vi "Actor Core.vi"(8 "error in":errorcluster, 11 "Game Engine in":refnum<class "Game Engine.lvclass">) -> (0 "error out":errorcluster, 3 "Actor out":refnum<class "Actor.lvclass">)   [LabVIEW 2017, in "Game Engine.lvlib" / "Game Engine.lvclass"]
doc: "(<B>Filename</B>: Actor Framework.lvlib:Actor.lvclass:Actor Core.vi)\n\nReceives messages to the actor, reacts to them, and initiates any error handling that may shut the actor down.\n\nDescendant classes may override this VI to append parallel tasks for the actor to complete while it handles messages. Overrides use the Call Parent Method node."
uses:
  Game Engine.lvclass
  <vilib>/ActorFramework/Actor/Actor.lvclass
  Simulated Screen Interface/Simulated Screen Interface/Simulated Screen Interface.lvclass
  C:/Program Files (x86)/National Instruments/LabVIEW 2017/vi.lib/ActorFramework/Actor/Actor.lvclass
  Simulated Game Pad Interface/Simulated Game Pad Interface.lvclass
  C:/Users/chris/Documents/GitHub/Tetris/RT Code/Abstract Game Pad Interface/Abstract Game Pad Interface.lvclass
  Simulated Screen Interface/Simulated Screen Interface Messages/Update Display Msg/Update Display Msg.lvclass
  C:/Users/chris/Documents/GitHub/Tetris/RT Code/Screen Interface/Screen Interface Messages/Display Game Board Msg/Display Game Board Msg.lvclass
  Game Engine.lvclass/Game Engine.ctl
  <vilib>/Platform/TimedLoop/XDataNode/timing_clust.ctl
  <vilib>/Platform/TimedLoop/XDataNode/nitl_modes.ctl
  <vilib>/Platform/TimedLoop/XDataNode/wakeup.ctl
  Error Handler/Error Handler/Error Handler.lvclass
  <vilib>/Platform/TimedLoop/XDataNode/XDataNode.xnode
  Abstract Game Pad Interface/Abstract Game Pad Interface.lvclass
  <vilib>/Platform/TimedLoop/XDataNode/XDNodeRunTimeDep.lvlib
  Hardware Game Pad Interface/Hardware Game Pad Interface.lvclass
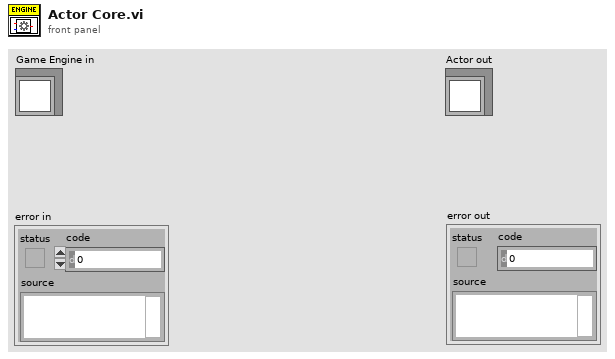
[diagram p1: front panel]
types:
  T1 = typedef "XDNodeRunTimeDep.lvlib/timing_clust.ctl" = cluster{"Expected End [f-1]":u64, "Actual End [f-1]":u64, "Finished Late? [f-1]":bool, "Expected End [i-1]":u64, "Actual End [i-1]":u64, "Finished Late? [i-1]":bool, "Expected Start [i]":u64, "Actual Start [i]":u64, "Expected Start [f]":u64, "Actual Start [f]":u64, "Source Name":string, "Structure Name":string, "Period":i64, "Deadline":i64, "Offset":i64, "Start":i64, "Priority":i32, "Timeout":i32, "Mode":T2, "Wakeup Reason":T3, "Error":errorcluster, "Source Type":string, "Secondary Source Type":string, "Global End Time":u64, "Global Start Time":u64, "Frame Duration":u64, "Iteration Duration":u64, "Assigned CPU":i32, "I/O Scan Engine Mode":u32}
  T2 = typedef "XDNodeRunTimeDep.lvlib/nitl_modes.ctl" = enum32{"No Change", "Process missed periods, maintain original phase", "Discard missed periods, maintain original phase", "Process missed periods, ignore original phase", "Discard missed periods, ignore original phase"}
  T3 = typedef "XDNodeRunTimeDep.lvlib/wakeup.ctl" = enum32{"Normal", "Aborted", "Asynchronous wakeup", "Timing source error", "Timed loop error", "Timeout"}
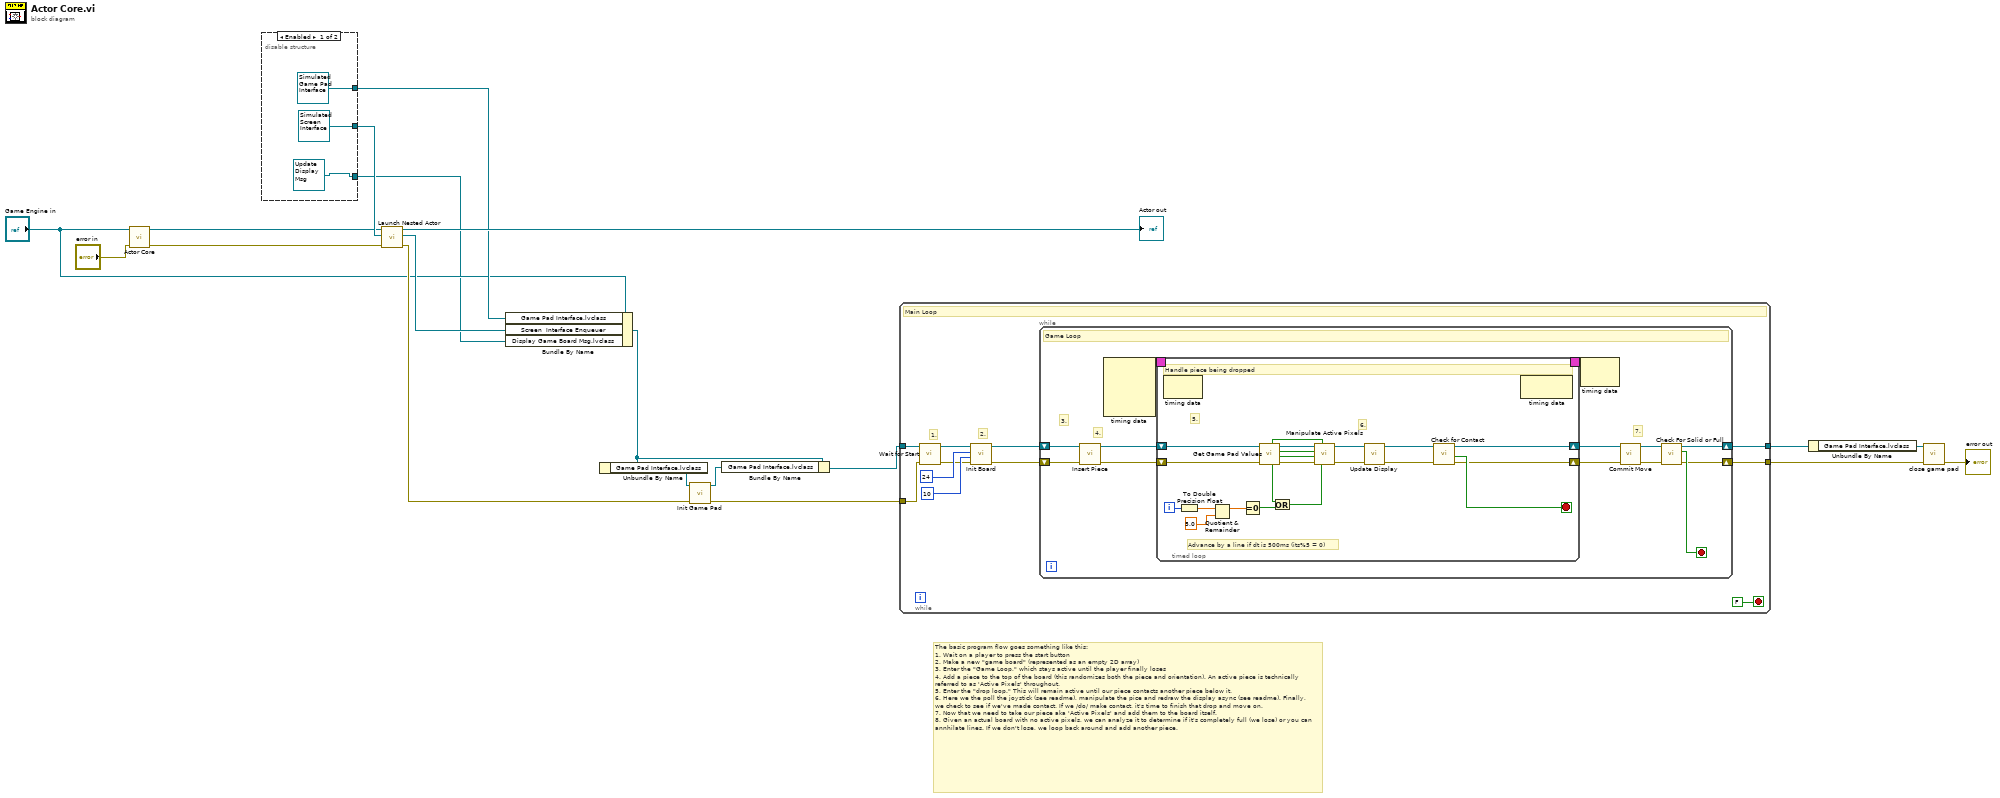
[diagram p0: block diagram]
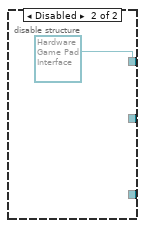
[diagram p2: hidden frame]
diagram:
  # "The basic program flow goes something like this:\n1. Wait on a player to press the start button\n2. Make a new \"game board\" (represented as an empty 2D array)\n3. Enter the \"Game Loop,\" which stays active until the player finally loses\n4. Add a piece to the top of the board (this randomizes both the piece and orientation). An active piece is technically referred to as 'Active Pixels' throughout.\n5. Enter the \"drop loop.\" This will remain active until our piece contacts another piece below it.\n6. Here we the poll the joystick (see readme), manipulate the pice and redraw the display async (see readme). Finally, we check to see if we've made contact. If we /do/ make contact, it's time to finish that drop and move on.\n7. Now that we need to take our piece aka 'Active Pixels' and add them to the board itself. \n8. Given an actual board with no active pixels, we can analyze it to determine if it's completely full (we lose) or you can annhilate lines. If we don't lose, we loop back around and add another piece."
  n1 = call-parent "Actor Core.vi"("error in"="error in", "Controller in"="Game Engine in") -> ("error out"=w3:errorcluster, "Actor out"=w6:refnum<class "Actor.lvclass">)  [unwired: 8 in]
  n2 = disable-structure shown="Enabled" {
    disable-tunnel: [refnum<class "Simulated Screen Interface.lvclass"> refnum ("Simulated Screen Interface.lvlib:Simulated Screen Interface.lvclass") w24] -> w19
    disable-tunnel: [refnum<class "Simulated Game Pad Interface.lvclass"> refnum ("Simulated Game Pad Interface.lvclass") refnum<class "Hardware Game Pad Interface.lvclass"> refnum ("Hardware Game Pad Interface.lvclass")] -> w15
    disable-tunnel: [refnum<class "Update Display Msg.lvclass"> refnum ("Simulated Screen Interface.lvlib:Update Display Msg.lvclass") w23] -> w1
    frame Enabled {
    }
    frame Disabled {
    }
  }
  n3 = call <vilib>:"Launch Nested Actor.vi"("error in (no error)"=w3, "Nested Actor"=w19, "Caller Actor in"=w6) -> ("error out"=w16:errorcluster, "Nested Actor's Enqueuer"=w18:refnum<class "Message Enqueuer.lvclass">, "Caller Actor out"=→"Actor out":refnum<class "Actor.lvclass">)  [unwired: 6 in]
  n4 = Bundle By Name(cluster="Game Engine in", "Game Pad Interface.lvclass"=w15, "Screen  Interface Enqueuer"=w18, "Display Game Board Msg.lvclass"=w1) -> (w13:refnum<class "Game Engine.lvclass">)
  n5 = Unbundle By Name(w13) -> ("Game Pad Interface.lvclass"=w14:refnum<class "Abstract Game Pad Interface.lvclass">)
  n6 = call-dynamic "Init Game Pad.vi"("error in (no error)"=w16, "Abstract Game Pad Interface in"=w14) -> ("error out"=w10:errorcluster, "Abstract Game Pad Interface out"=w12:refnum<class "Abstract Game Pad Interface.lvclass">)  [unwired: 8 in]
  n7 = Bundle By Name(cluster=w13, "Game Pad Interface.lvclass"=w12) -> (w11:refnum<class "Game Engine.lvclass">)
  n8 = while {
    tunnel: w11 -> [w32]
    tunnel: [w28] -> w7
    tunnel: [w27] -> w9
    tunnel: w10 -> [w26]
    stop <- FALSE stop-if-true
    # "2."
    # "1."
    # "Main Loop"
    n9 = call "Wait for Start.vi"("error in (no error)"=w26, "Game Engine in"=w32) -> ("error out"=w30:errorcluster, "Game Engine out"=w31:refnum<class "Game Engine.lvclass">)  [unwired: 8 in]
    n10 = call "Init Board.vi"("error in (no error)"=w30, "Columns"=u8 10, "Rows"=u8 24, "Game Engine in"=w31) -> ("error out"=w33:errorcluster, "Game Engine out"=w34:refnum<class "Game Engine.lvclass">)  [unwired: 6 in]
    n11 = while {
      shift-right: [w37] -> w27
      shift-left: w34 -> [w47]
      shift-right: [w38] -> w28
      shift-left: w33 -> [w46]
      stop <- w39 stop-if-true
      # "7."
      # "4."
      # "3."
      # "Game Loop"
      n12 = call "Insert Piece.vi"("error in (no error)"=w46, "Game Engine in"=w47) -> ("error out"=w44:errorcluster, "Game Engine out"=w45:refnum<class "Game Engine.lvclass">)  [unwired: 8 in]
      n13 = node-c288() -> (w49:T1)  [unwired: 4 in]
      n14 = timed-loop {
        timing: w49 -> [_]
        timing-out: [_] -> w48
        shift-right: [w50] -> w43
        shift-left: w45 -> [w57]
        shift-right: [w51] -> w42
        shift-left: w44 -> [w56]
        i -> [w69]
        stop <- w70 stop-if-true
        # "6."
        # "5."
        # "Advance by a line if dt is 500ms (its%5 = 0)"
        # "Handle piece being dropped"
        n15 = node-c288() -> ()  [unwired: 1 in, 1 out]
        n16 = To Double Precision Float(number=w69) -> (double precision float=w68:dbl)
        n17 = Quotient & Remainder(x=w68, y=5.0) -> (x-y*floor(x/y)=w66:dbl)  [unwired: 1 out]
        n18 = Equal To 0?(x=w66) -> (x = 0?=w65:bool)
        n19 = call "Get Game Pad Values.vi"("error in (no error)"=w56, "Game Engine in"=w57) -> ("error out"=w60:errorcluster, "Right"=w61:bool, "Left"=w62:bool, "Game Engine out"=w59:refnum<class "Game Engine.lvclass">, "Down"=w64:bool, "Rotate"=w58:bool)  [unwired: 3 in, 1 out]
        n20 = Or(x=w64, y=w65) -> (x .or. y?=w63:bool)
        n21 = call "Manipulate Active Pixels.vi"("Advance Line"=w63, "Rotate"=w58, "error in (no error)"=w60, "Right"=w61, "Left"=w62, "Game Engine in"=w59) -> ("error out"=w54:errorcluster, "Game Engine out"=w55:refnum<class "Game Engine.lvclass">)  [unwired: 4 in]
        n22 = call "Update Display.vi"("error in (no error)"=w54, "Game Engine in"=w55) -> ("error out"=w53:errorcluster, "Game Engine out"=w52:refnum<class "Game Engine.lvclass">)  [unwired: 8 in]
        n23 = call "Check for Contact.vi"("error in (no error)"=w53, "Game Engine in"=w52) -> ("error out"=w51:errorcluster, "Contact"=w70:bool, "Game Engine out"=w50:refnum<class "Game Engine.lvclass">)  [unwired: 7 in]
        n24 = node-c288() -> ()  [unwired: 1 in, 1 out]
      }
      n25 = node-c288(w48) -> ()  [unwired: 1 out]
      n26 = call "Commit Move.vi"("error in (no error)"=w42, "Game Engine in"=w43) -> ("error out"=w40:errorcluster, "Game Engine out"=w41:refnum<class "Game Engine.lvclass">)  [unwired: 8 in]
      n27 = call "Check For Solid or Full.vi"("error in (no error)"=w40, "Game Engine in"=w41) -> ("error out"=w38:errorcluster, "Game Over"=w39:bool, "Game Engine out"=w37:refnum<class "Game Engine.lvclass">)  [unwired: 7 in]
    }
  }
  n28 = Unbundle By Name(w9) -> ("Game Pad Interface.lvclass"=w8:refnum<class "Abstract Game Pad Interface.lvclass">)
  n29 = call-dynamic "close game pad.vi"("error in (no error)"=w7, "Abstract Game Pad Interface in"=w8) -> ("error out"=→"error out":errorcluster)  [unwired: 8 in, 1 out]
